vi "EnqueueMessage(Single).vi"(6 "Priority Message? (F)":bool, 8 "error in (no error)":errorcluster, 9 "Message Data":variant, 10 "Message":string, 11 "Message Queue":refnum<queue>) -> (0 "error out":errorcluster, 3 "dup Message Queue":refnum<queue>)   [LabVIEW 2017, in "Client.lvlib" / "CommsFrameWork.lvlib"]
doc: "For a regular message, enqueue the message. For a priority message, enqueue it at the front of the queue."
uses:
  CommsFrameWork.lvlib
  ServerLib/SubLibs/Message Queue/MessageCluster.ctl
  ServerLib/SubLibs/Message Queue/Message Queue.lvlib
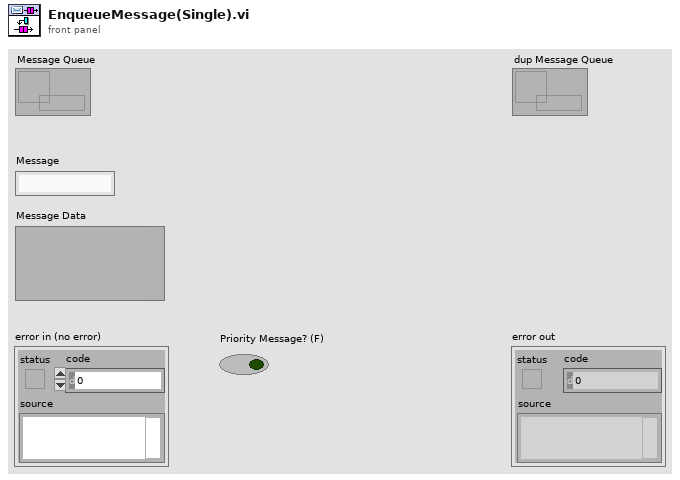
[diagram p1: front panel]
types:
  T1 = typedef "Server.lvlib/Message Queue.lvlib/MessageCluster.ctl" = cluster{"Message":string, "Message Data":variant}
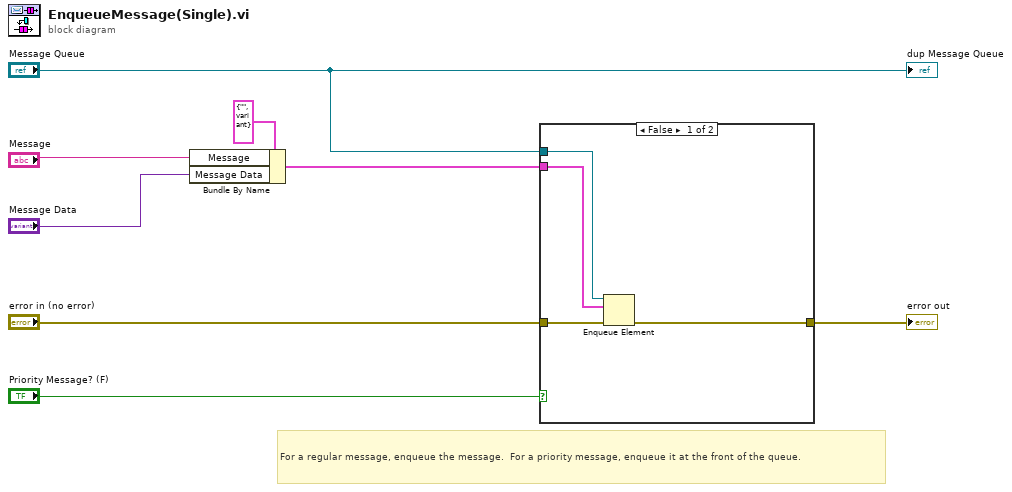
[diagram p0: block diagram]
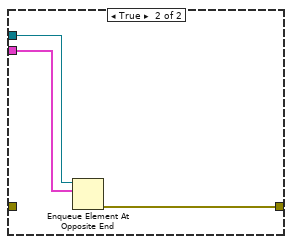
[diagram p2: hidden frame]
diagram:
  # "For a regular message, enqueue the message.  For a priority message, enqueue it at the front of the queue."
  n1 = Bundle By Name(cluster=T1 {"Message"="", "Message Data"=variant} ("Message Cluster"), "Message"="Message", "Message Data"="Message Data") -> (w2:T1)
  n2 = case shown="False" "Priority Message? (F)" {
    tunnel: [w12 w15] -> w4
    tunnel: "Message Queue" -> [w11 w14]
    tunnel: w2 -> [w10 w13]
    tunnel: "error in (no error)" -> [w9 _]
    frame False {
      n3 = Enqueue Element(queue=w11, element=w10, error in (no error)=w9) -> (error out=w12:errorcluster)  [unwired: 1 in, 2 out]
    }
    frame True {
      n4 = Enqueue Element At Opposite End(queue=w14, element=w13) -> (error out=w15:errorcluster)  [unwired: 2 in, 2 out]
    }
  }
  "error out" <- w4
  "dup Message Queue" <- "Message Queue"
